vi "IRQ Handler.vi"(8 "error in":errorcluster, 9 "IRQ(s) Asserted":i32[](array[numeric]), 10 "Timeout (ms)":i32, 11 "FPGA VI Reference In":refnum<k20>) -> (3 "IRQ occurred":bool=TRUE)   [LabVIEW 2014]
uses:
  <vilib>/Utility/error.llb/Error Cluster From Error Code.vi
  <vilib>/RVI Host/nirviSupport.llb/nirviErrorClusterFromErrorCode.vi
  <vilib>/rvi/errors/niLvFpgaAdjustHostInterfaceError.vi
  <vilib>/rvi/interface/nirviMethod/nirviMethod.xnode
  <vilib>/rvi/interface/nirviMethod/StockFPGA_InlinedMethodWaitForMultipleIRQ.vi
  <vilib>/FPGAPlugInAG/Dynamic/niLvFpga_WaitOnIrq_Dynamic.vi
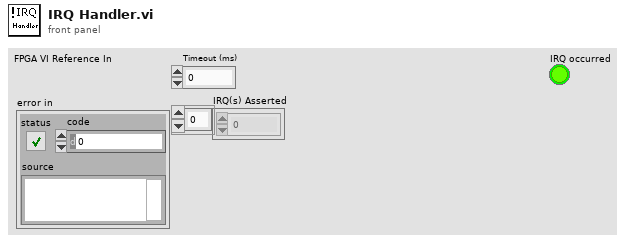
[diagram p1: front panel]
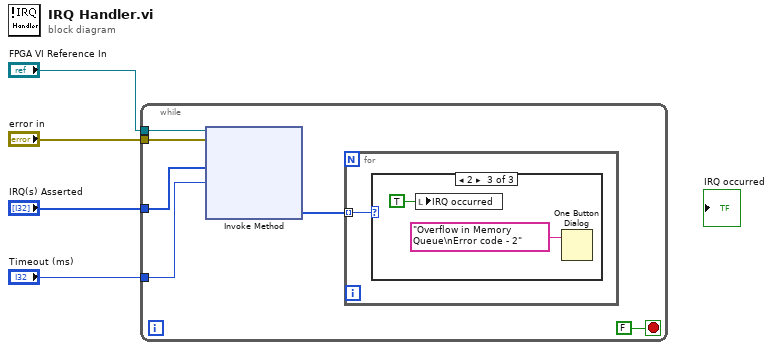
[diagram p0: block diagram]
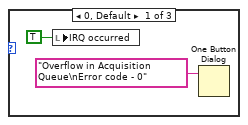
[diagram p2: hidden frame]
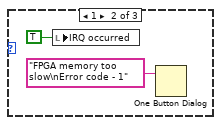
[diagram p3: hidden frame]
diagram:
  n1 = while {
    tunnel: "FPGA VI Reference In" -> [w10]
    tunnel: "error in" -> [w9]
    tunnel: "Timeout (ms)" -> [w8]
    tunnel: "IRQ(s) Asserted" -> [w6]
    stop <- FALSE stop-if-true
    n2 = xnode "Invoke Method"("FPGA VI Reference In"=w10, "error in"=w9, "IRQ Number(s)"=w6, "Timeout (ms)"=w8) -> ("IRQ(s) Asserted"=w7:i32[])  [unwired: 3 out]
    n3 = for {
      tunnel: w7 -> [w11] mode=indexing
      n4 = case shown="2" w11 {
        frame 0, Default {
          n5 = local write "IRQ occurred"(TRUE ("Boolean")) -> ()
          n6 = One Button Dialog(message="Overflow in Acquisition Queue\nError code - 0") -> ()  [unwired: 1 in, 1 out]
        }
        frame 1 {
          n7 = local write "IRQ occurred"(TRUE ("Boolean")) -> ()
          n8 = One Button Dialog(message="FPGA memory too slow\nError code - 1") -> ()  [unwired: 1 in, 1 out]
        }
        frame 2 {
          n9 = local write "IRQ occurred"(TRUE) -> ()
          n10 = One Button Dialog(message="Overflow in Memory Queue\nError code - 2") -> ()  [unwired: 1 in, 1 out]
        }
      }
    }
  }
